vi "Lev-Mar abx with 2D encoded Gaussian.vi"(4 "fit type":u16, 5 "Fit this coeff?":bool[](array[boolean]), 6 "derivative":T1(ring), 7 "code":dbl format="%.3f", 8 "Standard Deviation":dbl[](array[numeric]) format="%.2f", 9 "Coefficients":dbl[](array[numeric]) format="%.2f", 10 "Y":dbl[](array[numeric]) format="%.2f", 11 "X":dbl[](array[numeric]) format="%.2f") -> (0 "chiSqr":dbl format="%.2f", 1 "Beta":dbl[](array[numeric]) format="%.2f", 3 "Alpha":dbl[][](array[numeric]) format="%.2f")   [LabVIEW 2011]
doc: "This subprogram is derived from a subprogram contained in the National Instruments LabView advanced analysis library. The original subprogram is copyright National Instruments."
panel:
  # "Lev-Mar\nabx"
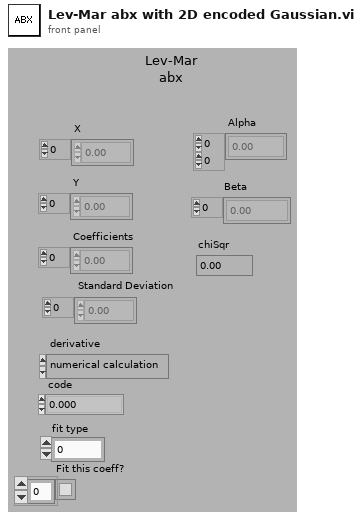
[diagram p1: front panel]
types:
  T1 = enum32{"numerical calculation", "formula calculation"}
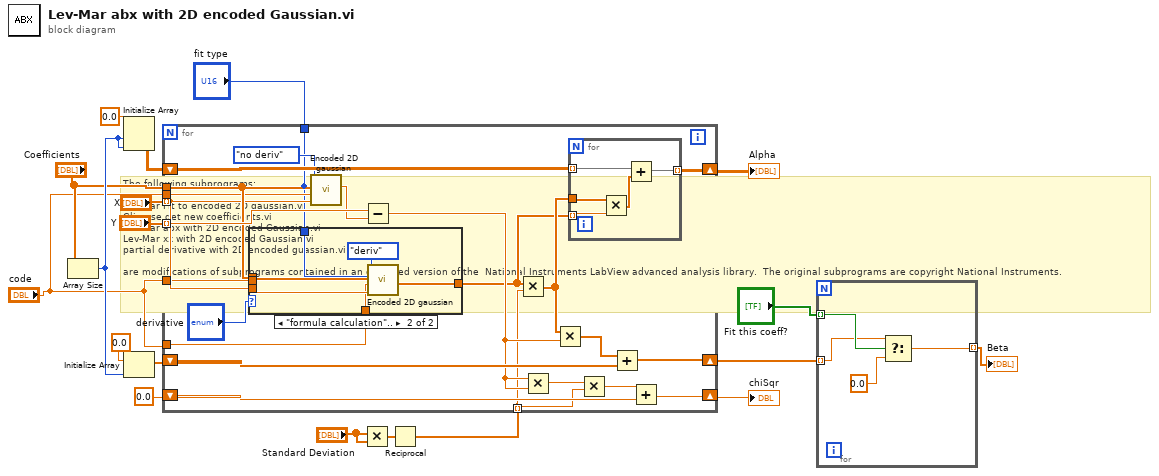
[diagram p0: block diagram]
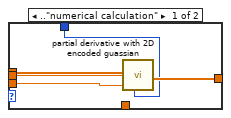
[diagram p2: hidden frame]
diagram:
  # "The following subprograms:\n\nLev-Mar Fit to encoded 2D gaussian.vi\nGlimpse get new coefficients.vi\nLev-Mar abx with 2D encoded Gaussian.vi\nLev-Mar xx with 2D encoded Gaussian.vi\npartial derivative with 2D encoded guassian.vi\n\nare modifications of subprograms contained in an outdated version of the  National Instruments LabView advanced analysis library.  The original subprograms are copyright National Instruments."
  n1 = Array Size(array="Coefficients") -> (size(s)=w17:i32)
  n2 = Initialize Array(0.0, w17, w17) -> (w15:dbl[][])
  n3 = Initialize Array(0.0, w17) -> (w16:dbl[])
  n4 = Multiply(x="Standard Deviation", y="Standard Deviation") -> (x*y=w8:dbl[])
  n5 = Reciprocal(x=w8) -> (1/x=w6:dbl[])
  n6 = for {
    tunnel: "X" -> [w30] mode=indexing
    shift-right: [w37] -> w2
    shift-left: w16 -> [w39]
    shift-right: [w34] -> w11
    shift-left: w15 -> [w35]
    shift-right: [w33] -> w7
    shift-left: 0.0 -> [w41]
    tunnel: "Y" -> [w40] mode=indexing
    tunnel: "Coefficients" -> [w31]
    tunnel: w6 -> [w25] mode=indexing
    tunnel: "code" -> [w23]
    tunnel: "code" -> [w22]
    tunnel: "code" -> [w21]
    tunnel: "fit type" -> [w20]
    n7 = case shown="\"formula calculation\".." "derivative" {
      tunnel: [w45 w53] -> w24
      tunnel: w31 -> [w47 w52]
      tunnel: w30 -> [w46 w51]
      tunnel: w23 -> [_ w49]
      tunnel: w21 -> [w44 _]
      tunnel: w20 -> [w43 w48]
      frame .."numerical calculation" {
        n8 = call "partial derivative with 2D encoded guassian.vi"("Coefficients"=w47, "code"=w44, "x"=w46, "fit type"=w43) -> ("Partial Derivative"=w45:dbl[])  [unwired: 3 out]
      }
      frame "formula calculation".. {
        n9 = call "Encoded 2D gaussian.vi"("Coefficients"=w52, "X"=w51, "code"=w49, "fit type"=w48, "Flag"=enum16{"no deriv", "deriv"}."deriv") -> ("Derivatives"=w53:dbl[])  [unwired: 4 out]
      }
    }
    n10 = call "Encoded 2D gaussian.vi"("Coefficients"=w31, "X"=w30, "code"=w22, "fit type"=w20, "Flag"=enum16{"no deriv", "deriv"}."no deriv") -> ("Y"=w32:dbl)  [unwired: 4 out]
    n11 = Subtract(x=w40, y=w32) -> (x-y=w36:dbl)
    n12 = Multiply(x=w24, y=w25) -> (x*y=w27:dbl[])
    n13 = Multiply(x=w36, y=w36) -> (x*y=w42:dbl)
    n14 = Multiply(x=w27, y=w36) -> (x*y=w38:dbl[])
    n15 = for {
      tunnel: w27 -> [w58]
      tunnel: w35 -> [w57] mode=indexing
      tunnel: [w55] -> w34 mode=indexing
      tunnel: w24 -> [w54] mode=indexing
      n16 = Multiply(x=w58, y=w54) -> (x*y=w56:dbl[])
      n17 = Add(x=w57, y=w56) -> (x+y=w55:dbl[])
    }
    n18 = Multiply(x=w42, y=w25) -> (x*y=w26:dbl)
    n19 = Add(x=w38, y=w39) -> (x+y=w37:dbl[])
    n20 = Add(x=w26, y=w41) -> (x+y=w33:dbl)
  }
  "Alpha" <- w11
  "chiSqr" <- w7
  n21 = for {
    tunnel: "Fit this coeff?" -> [w62] mode=indexing
    tunnel: w2 -> [w61] mode=indexing
    tunnel: [w60] -> w1 mode=indexing
    n22 = Select(t=w61, s=w62, f=0.0) -> (s? t:f=w60:dbl)
  }
  "Beta" <- w1
